vi "SLSC Create Commands Section.vi"(0 "Parent Ref in":T1 format="%.0x", 1 "GUID Command Page":string, 2 "GUID Command Channel Page":string, 5 "Command Channel":string, 7 "Physical Channel":string, 9 "commands":T2[](array[typedef]), 11 "error in (no error)":errorcluster, 12 "SLSCChannelPath":string, 13 "Documentation":string) -> (4 "Parent Ref out":T1 format="%.0x", 15 "error out":errorcluster)   [LabVIEW 2015, in "SLSC CD System Explorer.lvlib"]
uses:
  SLSC CD System Explorer.lvlib
  SLSC EDS API/JSON parsing/command.ctl
  <vilib>/NI Veristand/Custom Device API/Custom Device Item Ref.ctl
  <vilib>/NI VeriStand/Custom Device API/Custom Device API.lvlib
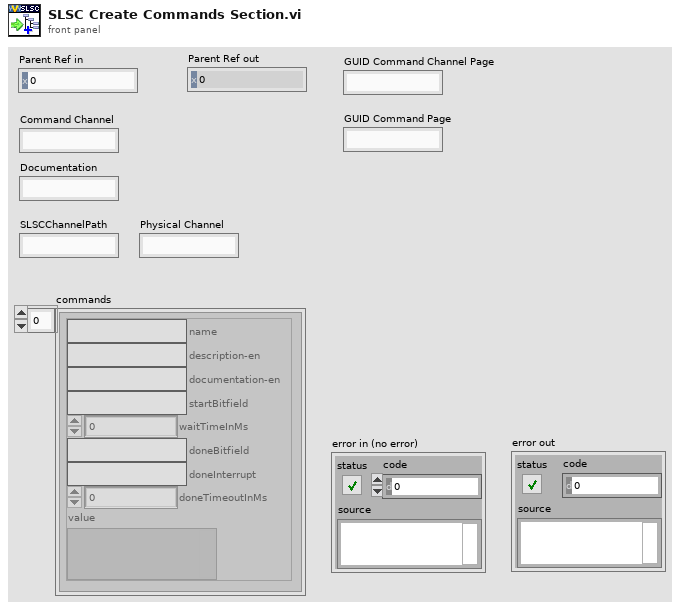
[diagram p1: front panel]
types:
  T1 = typedef "Custom Device API.lvlib/Custom Device Item Ref.ctl" = u64
  T2 = typedef "command.ctl" = cluster{"name":string, "description-en":string, "documentation-en":string, "startBitfield":string, "waitTimeInMs":i32, "doneBitfield":string, "doneInterrupt":string, "doneTimeoutInMs":i32, "value":variant}
  T3 = typedef "Custom Device API.lvlib/Custom Device Channel.ctl" = cluster{"Type":T4, "Units":string, "Default Value":dbl, "Faultable":bool, "Scalable":bool}
  T4 = typedef "Custom Device API.lvlib/Custom Device Channel Type.ctl" = enum16{"Input", "Output"}
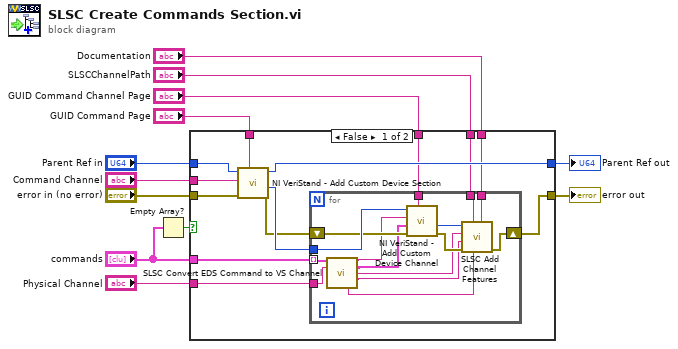
[diagram p0: block diagram]
diagram:
  n1 = Empty Array?(array="commands") -> (empty?=w12:bool)
  n2 = case shown="False" w12 {
    tunnel: [w25 w41] -> w1
    tunnel: [w24 w42] -> w2
    tunnel: "Parent Ref in" -> [w23 w42]
    tunnel: "error in (no error)" -> [w22 w41]
    tunnel: "Documentation" -> [w21 _]
    tunnel: "GUID Command Channel Page" -> [w20 _]
    tunnel: "SLSCChannelPath" -> [w19 _]
    tunnel: "Physical Channel" -> [w18 _]
    tunnel: "GUID Command Page" -> [w17 _]
    tunnel: "Command Channel" -> [w16 _]
    tunnel: "commands" -> [w15 _]
    frame False {
      n3 = call <vilib>:"NI VeriStand - Add Custom Device Section.vi"("GUID (Default Section)"=w17, "error in (no error)"=w22, "Section Name"=w16, "Parent Ref in"=w23) -> ("error out"=w13:errorcluster, "Section Ptr"=w14:T1, "Parent Ref out"=w24:T1)  [unwired: 4 in, 1 out]
      n4 = for {
        tunnel: w14 -> [w38]
        shift-right: [w36] -> w25
        shift-left: w13 -> [w37]
        tunnel: w15 -> [w32] mode=indexing
        tunnel: w20 -> [w35]
        tunnel: w19 -> [w34]
        tunnel: w21 -> [w33]
        tunnel: w18 -> [w31]
        n5 = call "SLSC Convert EDS Command to VS Channel.vi"("command"=w32, "Physical Channel"=w31) -> ("name"=w30:string, "Channel"=w29:T3, "SLSC Command Name"=w28:string, "documentation-en"=w27:string, "description-en"=w26:string)  [unwired: 9 in]
        n6 = call <vilib>:"NI VeriStand - Add Custom Device Channel.vi"("GUID (Default Channel)"=w35, "error in (no error)"=w37, "Channel"=w29, "Channel Name"=w30, "Parent Ref in"=w38) -> ("error out"=w39:errorcluster, "Channel Ref"=w40:T1)  [unwired: 3 in, 2 out]
        n7 = call "SLSC Add Channel Features.vi"("Documentation"=w33, "description-en"=w26, "SLSCChannelPath"=w34, "error in (no error)"=w39, "documentation-en"=w27, "SLSC Command Name"=w28, "Channel Ref"=w40) -> ("error out"=w36:errorcluster)  [unwired: 4 in]
      }
    }
    frame True {
    }
  }
  "Parent Ref out" <- w2
  "error out" <- w1
